vi "ExcelSaveData.vi"(8 "error in (no error)":errorcluster, 9 "data":string[](array[string]), 11 "template (empty)":path) -> (0 "error out":errorcluster)   [LabVIEW 2016]
uses:
  <vilib>/addons/_office/excel.llb/Excel Easy Table (str).vi
  <vilib>/Utility/NIReport.llb/NI_report.lvclass
  <vilib>/Utility/NIReport.llb/Excel/NI_Excel.lvclass
  <vilib>/addons/_office/NI_ReportGenerationToolkit.lvlib
panel:
  out "position (Excel)":cluster{"row":i32, "column":i32}
  in  "window state (normal)":T1(ring)=enum."no change"
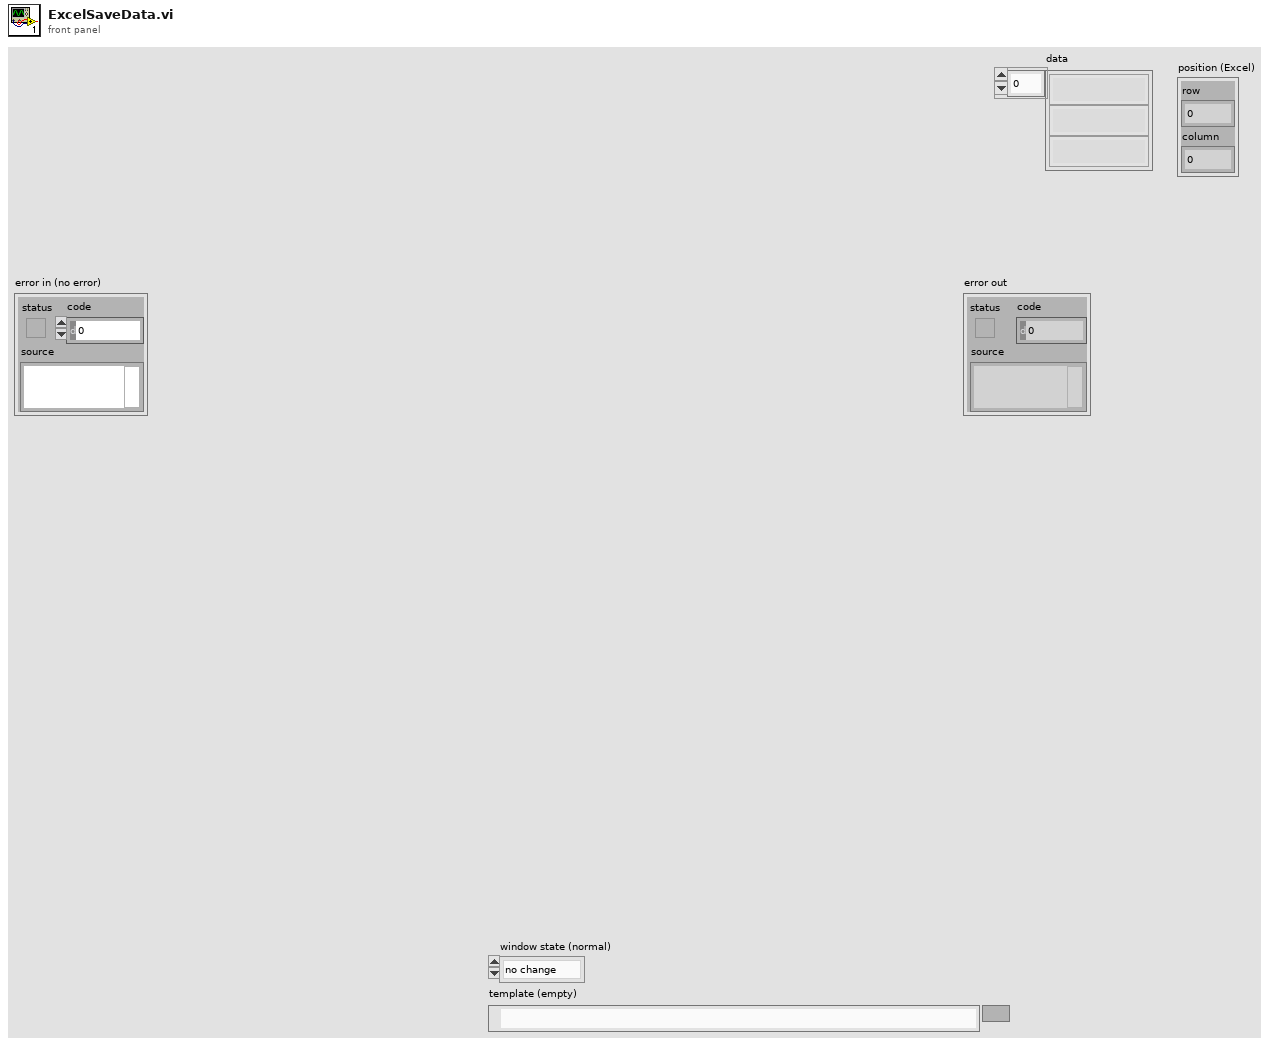
[diagram p1: front panel]
types:
  T1 = enum16{"maximized", "minimized", "normal", "no change"}
  T2 = enum16{"Standard Report", "HTML", "Word", "Excel"}
  T3 = cluster{"position (Excel)":cluster{"row":i32, "column":i32}, "name (Excel)":string, "bookmark (Word)":string}
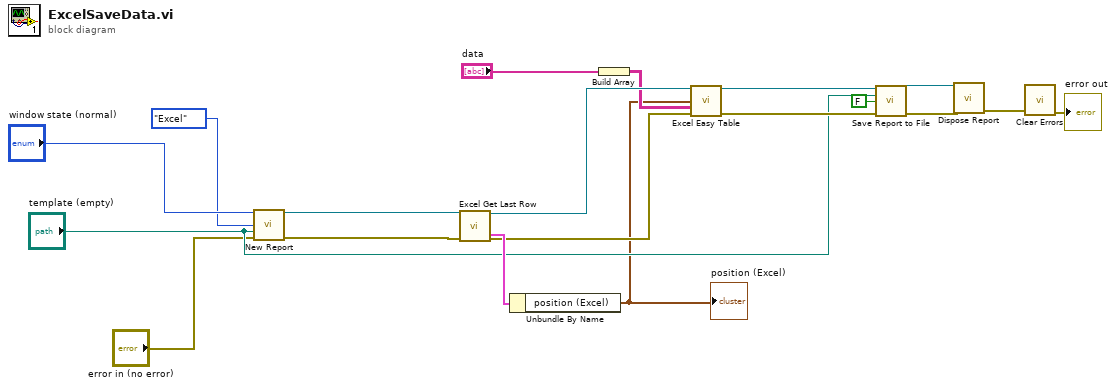
[diagram p0: block diagram]
diagram:
  n1 = call <vilib>:"New Report.vi"("window state (normal)"="window state (normal)", "report type"=T2."Excel", "template (empty)"="template (empty)", "error in (no error)"="error in (no error)") -> ("report out"=w17:refnum<class "NI_report.lvclass">, "error out"=w18:errorcluster)  [unwired: 10 in]
  n2 = call <vilib>:"Excel Get Last Row.vi"("report in"=w17, "error in (no error)"=w18) -> ("report out"=w14:refnum<class "NI_report.lvclass">, "MS Office parameters out"=w16:T3, "error out"=w13:errorcluster)  [unwired: 11 in]
  n3 = Unbundle By Name(w16) -> ("position (Excel)"=w5:cluster{"row":i32, "column":i32})
  "position (Excel)" <- w5
  n4 = Build Array("data") -> (w11:string[][])
  n5 = call-poly <vilib>:"Excel Easy Table.vi"("report in"=w14, "start (0, 0)"=w5, "text data"=w11, "error in (no error)"=w13) -> ("report out"=w10:refnum<class "NI_report.lvclass">, "error out"=w9:errorcluster)  [unwired: 7 in, 3 out]
  n6 = call-dynamic "Save Report to File.vi"("report in"=w10, "report file path"="template (empty)", "prompt to replace? (F)"=FALSE, "error in (no error)"=w9) -> ("report out"=w7:refnum<class "NI_report.lvclass">, "error out"=w8:errorcluster)  [unwired: 10 in]
  n7 = call-dynamic "Dispose Report.vi"("report in"=w7, "error in (no error)"=w8) -> ("error out"=w4:errorcluster)  [unwired: 13 in]
  n8 = call <vilib>:"Clear Errors.vi"("error in (no error)"=w4) -> ("error out"=→"error out":errorcluster)  [unwired: 5 in, 1 out]
